vi "Read Run Indefinitely.vi"(8 "error in (no error)":errorcluster, 11 "Measurement UI in":refnum<class "Measurement UI.lvclass">) -> (0 "error out":errorcluster, 2 "Run Indefinitely":refnum<vi>, 3 "Measurement UI out":refnum<class "Measurement UI.lvclass">)   [LabVIEW 2016, in "Measurement UI.lvlib" / "Measurement UI.lvclass"]
uses:
  Measurement UI.lvclass
  Measurement UI.lvclass/Measurement UI.ctl
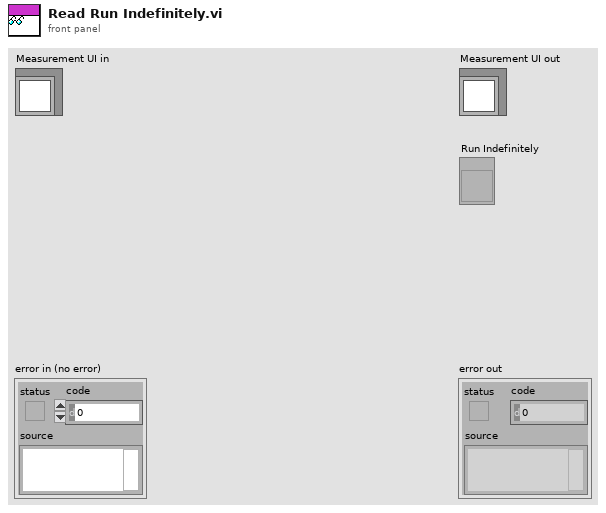
[diagram p1: front panel]
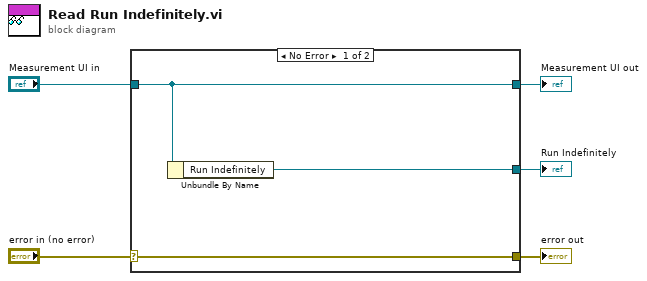
[diagram p0: block diagram]
diagram:
  n1 = case shown="No Error" "error in (no error)" {
    selector: "error in (no error)" -> [w8 w9]
    tunnel: [w8 w9] -> w4
    tunnel: [w7 w10] -> w2
    tunnel: "Measurement UI in" -> [w7 w10]
    tunnel: [w6 _] -> w1
    frame No Error {
      n2 = Unbundle By Name(w7) -> ("Run Indefinitely"=w6:refnum<vi>)
    }
    frame Error {
    }
  }
  "error out" <- w4
  "Measurement UI out" <- w2
  "Run Indefinitely" <- w1
